vi "OpenCamera.vi"(7 "error in (no error)":errorcluster, 10 "cameraName":string) -> (0 "error out":errorcluster, 2 "output":cluster{"Model":string, "Camera ID":string}, 3 "hCam out":i16)   [LabVIEW 2021]
panel:
  in  "output in":cluster{"Model":string, "Camera ID":string}
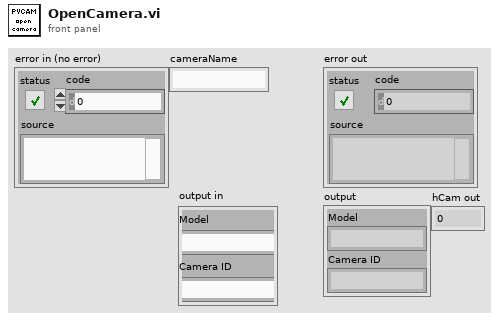
[diagram p1: front panel]
types:
  T1 = enum16{"ATTR_CURRENT", "ATTR_COUNT", "ATTR_TYPE", "ATTR_MIN", "ATTR_MAX", "ATTR_DEFAULT", "ATTR_INCREMENT", "ATTR_ACCESS", "ATTR_AVAIL"}
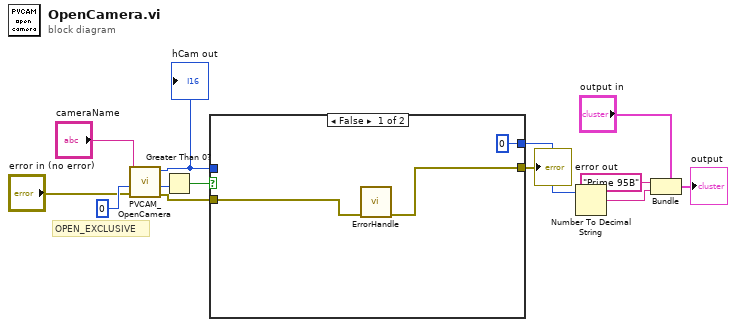
[diagram p0: block diagram]
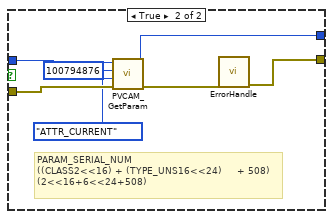
[diagram p2: hidden frame]
diagram:
  # "OPEN_EXCLUSIVE"
  n1 = call "PVCAM_OpenCamera.vi"("error in (no error)"="error in (no error)", "mode"=i16 0, "cameraName"="cameraName") -> ("error out"=w7:errorcluster, "return out"=w10:i16, "hCam out"=w8:i16)  [unwired: 6 in]
  "hCam out" <- w8
  n2 = Greater Than 0?(x=w10) -> (x > 0?=w9:bool)
  n3 = case shown="False" w9 {
    tunnel: w8 -> [_ w23]
    tunnel: w7 -> [w16 w22]
    tunnel: [w15 w17] -> w6
    tunnel: [i16 0 ("param_value") w19] -> w4
    frame False {
      n4 = call "ErrorHandle.vi"("error in (no error)"=w16) -> ("error in (no error) 2"=w15:errorcluster)  [unwired: 10 in]
    }
    frame True {
      # "PARAM_SERIAL_NUM\n((CLASS2<<16) + (TYPE_UNS16<<24)     + 508)\n(2<<16+6<<24+508)"
      n5 = call "PVCAM_GetParam.vi"("error in (no error)"=w22, "param_attrib"=T1."ATTR_CURRENT", "param_id"=u32 100794876, "hCam"=w23) -> ("error out"=w18:errorcluster, "param_value"=w19:i16)  [unwired: 5 in, 1 out]
      n6 = call "ErrorHandle.vi"("error in (no error)"=w18) -> ("error in (no error) 2"=w17:errorcluster)  [unwired: 10 in]
    }
  }
  "error out" <- w6
  n7 = Number To Decimal String(number=w4) -> (decimal integer string=w5:string)  [unwired: 1 in]
  n8 = Bundle(cluster="output in", "Model"="Prime 95B", "Camera ID"=w5) -> (→"output":cluster{"Model":string, "Camera ID":string})
